vi "Find Recorders.vi"() -> ()   [LabVIEW 2015]
uses:
  <vilib>/Instr/_visa.llb/VISA Find Search Mode.ctl
panel:
  out "Names":string[](array[string])
  out "find list":refnum<visa-resource-name>[](array[refnum])
  out "Error Out":errorcluster
  in  "Error In":errorcluster
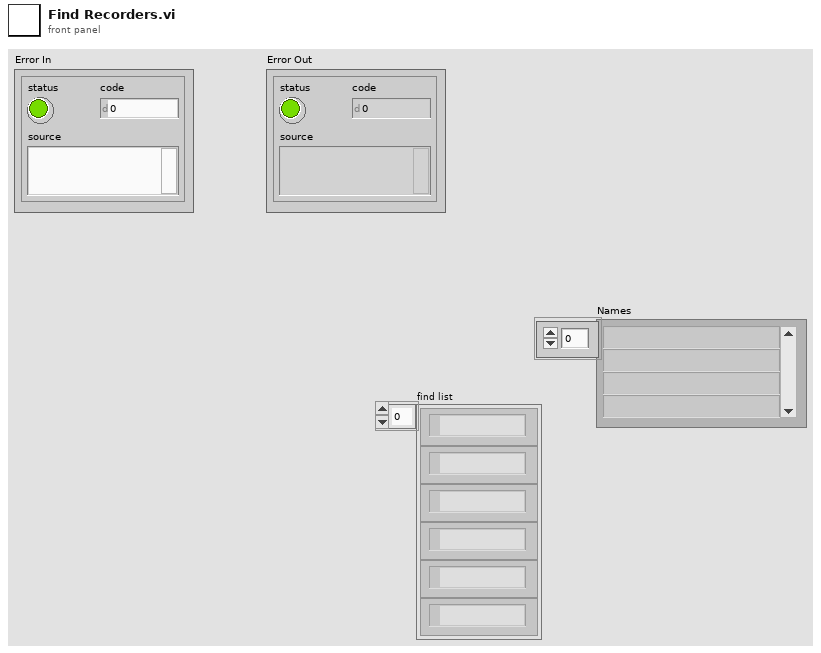
[diagram p1: front panel]
types:
  T1 = typedef "VISA Find Search Mode.ctl" = u32
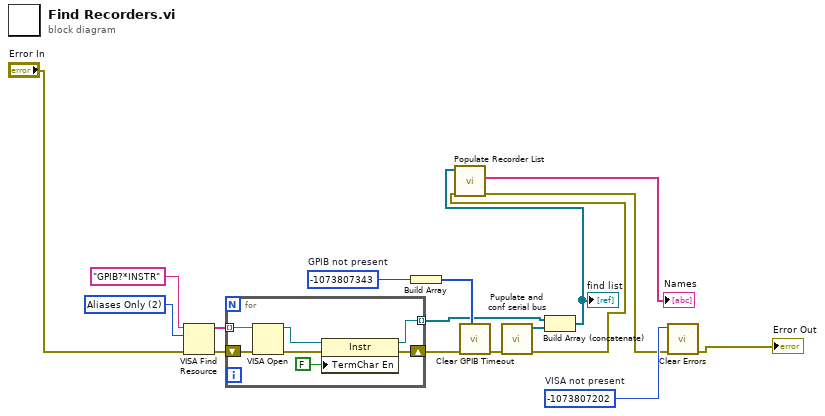
[diagram p0: block diagram]
diagram:
  w7 = -1073807202  # VISA not present
  w14 = -1073807343  # GPIB not present
  w16 = T1 2 items=["Canonical Names Only"=0, "Aliases Only"=2, "Include Matching Aliases"=3, "Include All Aliases"=4] ("Search Mode")
  n1 = VISA Find Resource(8:"Error In", 10:w16, 11:"GPIB?*INSTR" ("expression (\"?*\")")) -> (0:w11:errorcluster, 3:w9:string[])  [unwired: 1 out]
  n2 = for {
    shift-right: [w20] -> w10
    shift-left: w11 -> [w22]
    tunnel: w9 -> [w24] mode=indexing
    tunnel: [w19] -> w8 mode=indexing
    n3 = VISA Open(error in (no error)=w22, VISA resource name=w24) -> (VISA resource name=w23:refnum<visa-resource-name>, error out=w21:errorcluster)  [unwired: 3 in]
    n4 = property class="Instr"(reference=w23, error in=w21, "TermChar En"=FALSE ("Message Based Settings:Termination Character Enable")) -> (reference out=w19:refnum<visa-resource-name>, error out=w20:errorcluster)
  }
  n5 = Build Array(w14) -> (w13:i32[])
  n6 = call "Clear GPIB Timeout.vi"("Errors to skip"=w13, "error in (no error)"=w10) -> ("error out"=w12:errorcluster)  [unwired: 9 out]
  n7 = call "Pupulate and conf serial bus.vi"("Error In"=w12) -> ("Error Out"=w4:errorcluster, "Devices"=w15:refnum<visa-resource-name>[])  [unwired: 9 in]
  n8 = Build Array (concatenate)(w8, w15) -> (w3:refnum<visa-resource-name>[])
  "find list" <- w3
  n9 = call "Populate Recorder List.vi"("error in (no error)"=w4, "VISA Resourse Names"=w3) -> ("error out"=w2:errorcluster, "Names"=→"Names":string[])  [unwired: 7 in, 1 out]
  n10 = call <vilib>:"Clear Errors.vi"("error in (no error)"=w2, "specific error code to clear (0: all)"=w7) -> ("error out"=→"Error Out":errorcluster)  [unwired: 4 in, 1 out]
